vi "PSTRA-Init Reanalysis.vi"(0 "Path":path, 5 "PSTR Params":T31={"Stimulus"={"Ear"=enum."Right", "BW (oct)"=0.0, "Seed"=0, "Ramp (ms)"=0.0, "On time (ms)"=0.0, "Off time (ms)"=0.0, "Delay (ms)"=10000.0}, "FreqSeq"={"Min (kHz)"=0.0, "Max (kHz)"=0.0, "Step (oct)"=0.0}, "LevelSeq"={"Min (dB)"=0.0, "Max (dB)"=0.0, "Step (dB)"=0.0}, "Seq"={"Order"=enum."Sequential", "Averages"=0}, "Response"={"Grass gain"=0.0, "Window (ms)"=0.0}, "Hidden"={"Sample rate (Hz)"=0.0, "Nfft"=0, "save raw"=FALSE, "sep"=0.0, "Window"=enum."NONE"}, "RejThr"=0.0}) -> (4 "Data":T28, 8 "SCL":T27[](array[typedef]), 14 "Runtime out":T1 {"window" items=["None ", "Hanning", "Hamming", "Blackman-Harris", "Exact Blackman", "Blackman", "Flat Top", "4 Term B-Harris ", "7 Term B-Harris", "Low Sidelobe"]; "stimChan"."Filter"."Stages"."IIR Filter"."Forward Coefficients" format="%.4f"; "stimChan"."Filter"."Stages"."IIR Filter"."Reverse Coefficients" format="%.4f"})   [LabVIEW 2020]
uses:
  PSTR VIs/Typedefs/PSTR-Parameters.ctl
  PSTR VIs/Typedefs/PSTR-Stimulus Params.ctl
  Utility VIs/Type Defs/Left-Right ring.ctl
  PSTR VIs/Typedefs/PSTR-FreqSeq Params.ctl
  PSTR VIs/Typedefs/PSTR-LevelSeq Params.ctl
  PSTR VIs/Typedefs/PSTR-SeqParams.ctl
  PSTR VIs/Typedefs/PSTR-Response Params.ctl
  PSTR VIs/Typedefs/PSTR-Hidden Params.ctl
  PSTR VIs/Typedefs/PSTR-Window Shape.ctl
  PSTR VIs/Typedefs/PSTR-Data.ctl
  PSTR VIs/Typedefs/PSTR-Model Fit.ctl
  PSTR VIs/Typedefs/PSTR-Fit Parameters.ctl
  Typedefs/PSTR-SCL Element.ctl
  PSTR VIs/Typedefs/PSTR-Runtime Data.ctl
  Signal Synthesis VIs/Controls/Stimulus Channel (Full)/Full Stimulus Channel Data.ctl
  Signal Synthesis VIs/Controls/Waveform XCtl/Waveform Data.ctl
  Signal Synthesis VIs/Controls/Waveform XCtl/Waveform Enum.ctl
  Signal Synthesis VIs/Waveform VIs/Tone VIs/Tone Params.ctl
  Signal Synthesis VIs/Waveform VIs/Pulse Train VIs/Pulse Train Params.ctl
  Signal Synthesis VIs/Waveform VIs/Pulse Train VIs/Pulse Polarity.ctl
  Signal Synthesis VIs/Waveform VIs/Pulse Train VIs/PT-Continuous State.ctl
  Signal Synthesis VIs/Waveform VIs/Noise VIs/Noise Params.ctl
  Signal Synthesis VIs/Waveform VIs/File VIs/StimFile-Params.ctl
  Signal Synthesis VIs/Waveform VIs/FM Sweep VIs/FM Sweep Params.ctl
  Signal Synthesis VIs/Waveform VIs/Chirp Train VIs/Chirp Train.ctl
  Signal Synthesis VIs/Waveform VIs/Chirp Train VIs/Chirp Train Params.ctl
  Signal Synthesis VIs/Waveform VIs/Complex Tone VIs/CT-Params.ctl
  Signal Synthesis VIs/Waveform VIs/Complex Tone VIs/CT-Phase Enum.ctl
  Signal Synthesis VIs/Waveform VIs/Complex Tone VIs/CT-Runtime Data.ctl
  Signal Synthesis VIs/Waveform VIs/Moving Ripple VIs/Moving Ripple.ctl
  Signal Synthesis VIs/Waveform VIs/Moving Ripple VIs/Moving Ripple.Params.ctl
  Signal Synthesis VIs/Waveform VIs/Moving Ripple VIs/Moving Ripple.Data.ctl
  Signal Synthesis VIs/Controls/Advanced Filter XCtl/Filter Data.ctl
  Signal Synthesis VIs/Filter VIs/Filter-Bandwidth Units.ctl
  Signal Synthesis VIs/Controls/Burst XCtl/Burst Data.ctl
  Signal Synthesis VIs/Controls/Level XCtl/Level Data.ctl
  Signal Synthesis VIs/Controls/Level XCtl/Level Units.ctl
  Signal Synthesis VIs/Controls/Advanced Options XCtl/Advanced Stimulus Options.ctl
  Signal Synthesis VIs/Modulation VIs/SAM VIs/SAM Params.ctl
  Signal Synthesis VIs/Controls/Waveform XCtl/Waveform XCtl.xctl
  Signal Synthesis VIs/Controls/Advanced Filter XCtl/Advanced Filter XCtl.xctl
  Signal Synthesis VIs/Controls/Burst XCtl/Burst Control.xctl
  Signal Synthesis VIs/Controls/Level XCtl/Level XCtl.xctl
  Signal Synthesis VIs/Controls/Advanced Options XCtl/Advanced Stimulus Options.xctl
  Signal Synthesis VIs/Controls/Stimulus Channel (Full)/Stimulus Channel (Full).xctl
panel:
  # "NF x NL x 2 x Npts"
  # "NF x NL x Npts"
  # "NF x NL"
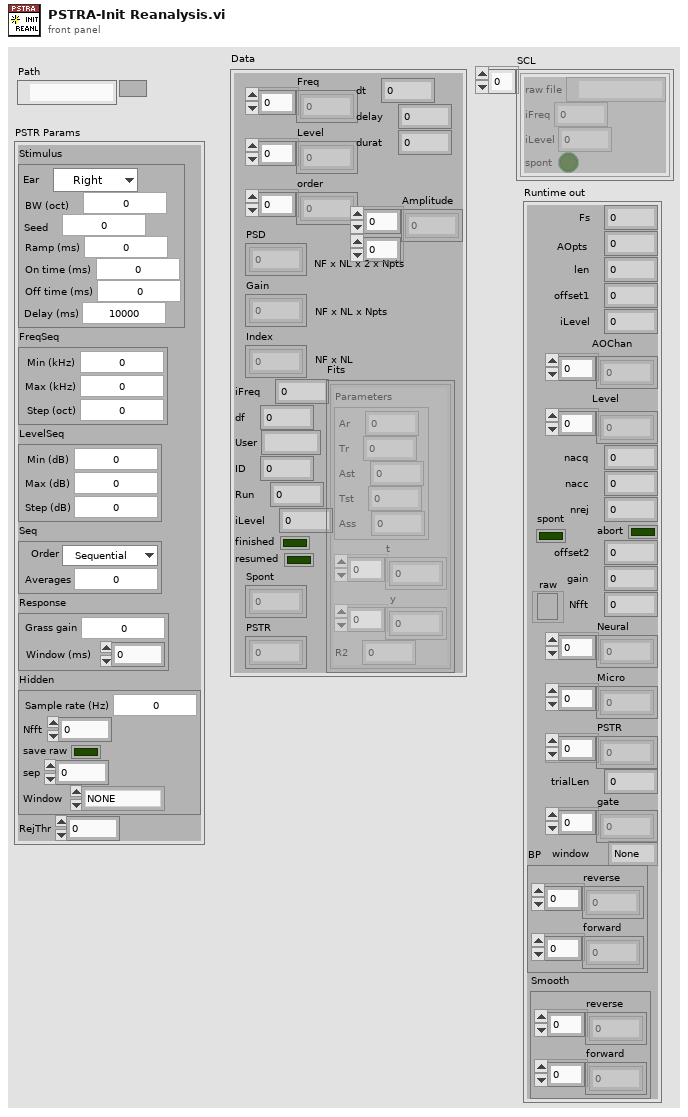
[diagram p1: front panel]
types:
  T1 = typedef "PSTR-Runtime Data.ctl" = cluster{"Fs":dbl, "AOpts":i32, "stimChan":T2, "len":i32, "offset1":i32, "iLevel":i32, "AOChan":i32[], "Level":dbl[], "nacc":i32, "nrej":i32, "nacq":i32, "abort":bool, "offset2":i32, "gain":dbl, "Nfft":i32, "Neural":dbl[], "Micro":dbl[], "raw":refnum<file>, "spont":bool, "PSTR":dbl[], "trialLen":i32, "gate":dbl[], "window":u16, "BP":cluster{"reverse":dbl[], "forward":dbl[]}, "Smooth":cluster{"reverse":dbl[], "forward":dbl[]}}
  T2 = typedef "Stimulus Channel (Full).xctl/Full Stimulus Channel Data.ctl" = cluster{"Waveform":T3, "Filter":T20, "Burst":T22, "Level":T23, "Name":string, "Advanced":T25, "SAM":T26}
  T3 = typedef "Waveform XCtl.xctl/Waveform Data.ctl" = cluster{"Type":T4, "Tone":T5, "Pulse Train":T6, "Noise":T9, "File":T10, "FMSweep":T11, "Chirp Train":T12, "Complex Tone":cluster{"Params":T14, "Data":T16}, "Moving Ripple":T17}
  T4 = typedef "Waveform Enum.ctl" = enum16{"OFF", "Tone", "Noise", "Pulse Train", "File", "FM Sweep", "Chirp Train", "Complex Tone", "FM Tone", "Moving Ripple"}
  T5 = typedef "Tone Params.ctl" = cluster{"Frequency (kHz)":dbl, "Last Freq":dbl, "Last Phase":dbl}
  T6 = typedef "Pulse Train Params.ctl" = cluster{"Pulse width (us)":dbl, "Pulse rate (Hz)":dbl, "Gap (ms)":dbl, "Polarity":T7, "PT State":T8, "Asynch":bool}
  T7 = typedef "Pulse Polarity.ctl" = enum16{"POS", "NEG", "POS-NEG", "NEG-POS"}
  T8 = typedef "PT-Continuous State.ctl" = cluster{"Template":dbl[], "Nperiod":i32, "Index":i32, "Pulse Rate (Hz)":dbl, "Phase (cycles)":dbl, "Noff":i32}
  T9 = typedef "Noise Params.ctl" = cluster{"InvFilt":bool, "Noise":dbl[], "CurPt":i32, "Aweight":bool, "Seed":i32, "afile":path}
  T10 = typedef "StimFile-Params.ctl" = cluster{"Filename":path, "Signal":dbl[], "Channel":i32, "stream":bool, "offset":i32, "nreps":i32, "loops":i32, "Randomize":bool, "order":i32[], "Seed":i32, "Tokens":i32}
  T11 = typedef "FM Sweep Params.ctl" = cluster{"Rate (oct/s)":dbl, "Fmin (Hz)":dbl, "Fmax (Hz)":dbl, "Ramp (ms)":dbl, "Linear":bool}
  T12 = typedef "Chirp Train.ctl" = cluster{"Params":T13, "Data":cluster{"WF":dbl[]}}
  T13 = typedef "Chirp Train Params.ctl" = cluster{"Fmin (kHz)":dbl, "Fmax (kHz)":dbl, "Compensate":bool, "Duration (ms)":dbl}
  T14 = typedef "CT-Params.ctl" = cluster{"F0 (Hz)":dbl, "Band":cluster{"Flow (Hz)":dbl, "Fhigh (Hz)":dbl}, "Phase":T15, "Min F0 (Hz)":dbl, "Max F0 (Hz)":dbl, "ContinRandPhase":bool, "Max peak factor":dbl, "Max mod depth":dbl, "MinHarmNum":i32, "MaxHarmNum":i32, "Level Mode":enum16{"per component", "overall rms"}, "% jitter":dbl}
  T15 = typedef "CT-Phase Enum.ctl" = enum16{"Cosine", "Random", "Alternating"}
  T16 = typedef "CT-Runtime Data.ctl" = cluster{"Ncomp":i32, "MinHarm":i32, "Phase":dbl[], "Amplitude":dbl[], "Npts/frame":i32, "Last F0":dbl, "Fmin":dbl, "Fmax":dbl, "Lslope":dbl, "randphase":bool, "overall rms":bool, "fmult":dbl[], "jittered":bool}
  T17 = typedef "Moving Ripple.ctl" = cluster{"Params":T18, "Data":T19}
  T18 = typedef "Moving Ripple.Params.ctl" = cluster{"Fmin":dbl, "Fmax":dbl, "Density":dbl, "Velocity":dbl, "Depth":dbl, "Phase":dbl, "Comp/oct":i32}
  T19 = typedef "Moving Ripple.Data.ctl" = cluster{"Freq":dbl[], "A":dbl[], "phase":dbl[], "Phase":dbl}
  T20 = typedef "Advanced Filter XCtl.xctl/Filter Data.ctl" = cluster{"Type":enum16{"Lowpass", "Highpass", "Bandpass", "Bandstop", "OFF"}, "CF (kHz)":dbl, "BW (kHz)":dbl, "Cascade":bool, "Quadrature":bool, "Scale Factor":dbl, "Stages":cluster{"IIR Filter":cluster{"filter structure":enum32{"IIR 2nd Order", "IIR 4th Order"}, "Reverse Coefficients":dbl[], "Forward Coefficients":dbl[]}, "State":dbl[]}[], "Class":enum16{"Elliptic", "Butterworth"}, "Order":i32, "BWUnits":T21}
  T21 = typedef "Filter-Bandwidth Units.ctl" = enum16{"Linear", "Octaves", "Min-Max"}
  T22 = typedef "Burst Control.xctl/Burst Data.ctl" = cluster{"Active":bool, "Delay (ms)":dbl, "Duration (ms)":dbl, "Ramp (ms)":dbl, "Rate (Hz)":dbl, "Trepeat (ms)":dbl, "Repeat":bool}
  T23 = typedef "Level XCtl.xctl/Level Data.ctl" = cluster{"Level":dbl, "Units":T24, "Max":dbl, "Multiplier":dbl, "Cal File":path, "Cal":cluster{"Freq (Hz)":dbl[], "Mag (dB SPL)":dbl[], "Phase (deg)":dbl[]}}
  T24 = typedef "Level Units.ctl" = enum16{"dB atten", "dB SPL", "dB re 1 Vrms", "dB V/Hz½", "mW", "dB HL", "Volts", "dB mW"}
  T25 = typedef "Advanced Stimulus Options.xctl/Advanced Stimulus Options.ctl" = cluster{"Rep Mask":string, "AltPol":bool, "Var":string, "Expr":string, "Persist":bool}
  T26 = typedef "SAM Params.ctl" = cluster{"Active":bool, "Frequency (Hz)":dbl, "Depth":dbl, "Init Phase (cycles)":dbl, "phase (degrees)":dbl, "Asynch":bool}
  T27 = typedef "PSTR-SCL Element.ctl" = cluster{"raw file":path, "iFreq":i32, "iLevel":i32, "spont":bool}
  T28 = typedef "PSTR-Data.ctl" = cluster{"Freq":dbl[], "Level":dbl[], "order":i32[], "PSD":dbl[][][][], "Gain":dbl[][][], "Index":dbl[][], "iFreq":i32, "df":dbl, "User":string, "ID":i32, "Run":i32, "iLevel":i32, "finished":bool, "resumed":bool, "Spont":dbl[][], "PSTR":dbl[][][], "dt":dbl, "delay":dbl, "durat":dbl, "Fits":T29[][], "Amplitude":dbl[][]}
  T29 = typedef "PSTR-Model Fit.ctl" = cluster{"Parameters":T30, "t":dbl[], "y":dbl[], "R2":dbl}
  T30 = typedef "PSTR-Fit Parameters.ctl" = cluster{"Ar":dbl, "Tr":dbl, "Ast":dbl, "Tst":dbl, "Ass":dbl}
  T31 = typedef "PSTR-Parameters.ctl" = cluster{"Stimulus":T32, "FreqSeq":T34, "LevelSeq":T35, "Seq":T36, "Response":T37, "Hidden":T38, "RejThr":dbl}
  T32 = typedef "PSTR-Stimulus Params.ctl" = cluster{"Ear":T33, "BW (oct)":dbl, "Seed":i32, "Ramp (ms)":dbl, "On time (ms)":dbl, "Off time (ms)":dbl, "Delay (ms)":dbl}
  T33 = typedef "Left-Right ring.ctl" = enum16{"Right", "Left"}
  T34 = typedef "PSTR-FreqSeq Params.ctl" = cluster{"Min (kHz)":dbl, "Max (kHz)":dbl, "Step (oct)":dbl}
  T35 = typedef "PSTR-LevelSeq Params.ctl" = cluster{"Min (dB)":dbl, "Max (dB)":dbl, "Step (dB)":dbl}
  T36 = typedef "PSTR-SeqParams.ctl" = cluster{"Order":enum16{"Sequential", "Random"}, "Averages":i32}
  T37 = typedef "PSTR-Response Params.ctl" = cluster{"Grass gain":dbl, "Window (ms)":dbl}
  T38 = typedef "PSTR-Hidden Params.ctl" = cluster{"Sample rate (Hz)":dbl, "Nfft":i32, "save raw":bool, "sep":dbl, "Window":T39}
  T39 = typedef "PSTR-Window Shape.ctl" = enum16{"NONE", "Hamming"}
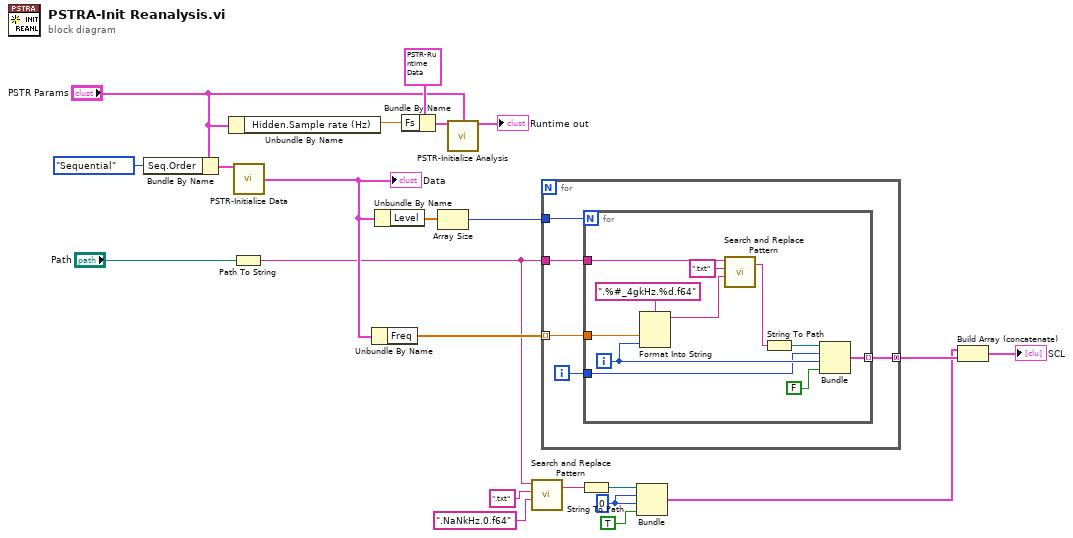
[diagram p0: block diagram]
diagram:
  w3 = 0
  n1 = Bundle By Name(cluster="PSTR Params", "Seq.Order"=enum16{"Sequential", "Random"}."Sequential") -> (w20:T31)
  n2 = Unbundle By Name("PSTR Params") -> ("Hidden.Sample rate (Hz)"=w10:dbl)
  n3 = Path To String(path="Path") -> (string=w8:string)
  n4 = call "PSTR-Initialize Data.vi"("PSTR Params"=w20) -> ("Data"=w15:T28)  [unwired: 13 in, 1 out]
  "Data" <- w15
  n5 = Unbundle By Name(w15) -> ("Freq"=w22:dbl[])
  n6 = Unbundle By Name(w15) -> ("Level"=w18:dbl[])
  n7 = Bundle By Name(cluster=T1 {"Fs"=0.0, "AOpts"=0, "stimChan"={"Waveform"={"Type"=enum."Tone", "Tone"={"Frequency (kHz)"=0.0, "Last Freq"=0.0, "Last Phase"=0.0}, "Pulse Train"={"Pulse width (us)"=0.0, "Pulse rate (Hz)"=0.0, "Gap (ms)"=0.0, "Polarity"=enum."POS", "PT State"={"Template"=[], "Nperiod"=0, "Index"=0, "Pulse Rate (Hz)"=0.0, "Phase (cycles)"=0.0, "Noff"=0}, "Asynch"=FALSE}, "Noise"={"InvFilt"=FALSE, "Noise"=[], "CurPt"=0, "Aweight"=FALSE, "Seed"=0, "afile"=path ""}, "File"={"Filename"=path "", "Signal"=[], "Channel"=0, "stream"=FALSE, "offset"=0, "nreps"=0, "loops"=0, "Randomize"=FALSE, "order"=[], "Seed"=0, "Tokens"=0}, "FMSweep"={"Rate (oct/s)"=0.0, "Fmin (Hz)"=0.0, "Fmax (Hz)"=0.0, "Ramp (ms)"=0.0, "Linear"=FALSE}, "Chirp Train"={"Params"={"Fmin (kHz)"=4.0, "Fmax (kHz)"=64.0, "Compensate"=FALSE, "Duration (ms)"=2.0}, "Data"={"WF"=[]}}, "Complex Tone"={"Params"={"F0 (Hz)"=0.0, "Band"={"Flow (Hz)"=0.0, "Fhigh (Hz)"=0.0}, "Phase"=enum."Cosine", "Min F0 (Hz)"=0.0, "Max F0 (Hz)"=0.0, "ContinRandPhase"=FALSE, "Max peak factor"=inf, "Max mod depth"=2.0, "MinHarmNum"=0, "MaxHarmNum"=0, "Level Mode"=enum."per component", "% jitter"=0.0}, "Data"={"Ncomp"=0, "MinHarm"=0, "Phase"=[], "Amplitude"=[], "Npts/frame"=0, "Last F0"=0.0, "Fmin"=0.0, "Fmax"=0.0, "Lslope"=0.0, "randphase"=FALSE, "overall rms"=FALSE, "fmult"=[], "jittered"=FALSE}}, "Moving Ripple"={"Params"={"Fmin"=0.0, "Fmax"=0.0, "Density"=0.0, "Velocity"=0.0, "Depth"=0.0, "Phase"=0.0, "Comp/oct"=0}, "Data"={"Freq"=[], "A"=[], "phase"=[], "Phase"=0.0}}}, "Filter"={"Type"=enum."Lowpass", "CF (kHz)"=0.0, "BW (kHz)"=0.0, "Cascade"=FALSE, "Quadrature"=FALSE, "Scale Factor"=0.0, "Stages"=[], "Class"=enum."Elliptic", "Order"=0, "BWUnits"=enum."Linear"}, "Burst"={"Active"=FALSE, "Delay (ms)"=0.0, "Duration (ms)"=0.0, "Ramp (ms)"=0.0, "Rate (Hz)"=0.0, "Trepeat (ms)"=0.0, "Repeat"=FALSE}, "Level"={"Level"=0.0, "Units"=enum."dB atten", "Max"=0.0, "Multiplier"=0.0, "Cal File"=path "", "Cal"={"Freq (Hz)"=[], "Mag (dB SPL)"=[], "Phase (deg)"=[]}}, "Name"="", "Advanced"={"Rep Mask"="", "AltPol"=FALSE, "Var"="", "Expr"="", "Persist"=FALSE}, "SAM"={"Active"=FALSE, "Frequency (Hz)"=0.0, "Depth"=0.0, "Init Phase (cycles)"=0.0, "phase (degrees)"=0.0, "Asynch"=FALSE}}, "len"=0, "offset1"=0, "iLevel"=0, "AOChan"=[], "Level"=[], "nacc"=0, "nrej"=0, "nacq"=0, "abort"=FALSE, "offset2"=0, "gain"=0.0, "Nfft"=0, "Neural"=[], "Micro"=[], "raw"=refnum, "spont"=FALSE, "PSTR"=[], "trialLen"=0, "gate"=[], "window"=0, "BP"={"reverse"=[], "forward"=[]}, "Smooth"={"reverse"=[], "forward"=[]}} ("Runtime in"), "Fs"=w10) -> (w11:T1)
  n8 = Array Size(array=w18) -> (size(s)=w17:i32)
  n9 = call "PSTR-Initialize Analysis.vi"("Runtime in"=w11, "PSTR Params"="PSTR Params") -> ("Runtime out"=→"Runtime out":T1)  [unwired: 12 in, 1 out]
  n10 = call <vilib>:"Search and Replace Pattern.vi"("string"=w8, "regular expression (\"\")"=".txt" ("regular expression (\"\")"), "replace string (\"\")"=".NaNkHz.0.f64" ("format string")) -> ("result string"=w4:string)  [unwired: 2 in, 1 out]
  n11 = for {
    tunnel: w22 -> [w27] mode=indexing
    tunnel: w8 -> [w26]
    tunnel: w17 -> [w25]
    tunnel: [w23] -> w16 mode=concatenating
    i -> [w24]
    n12 = for {
      N: w25 -> [_]
      tunnel: w27 -> [w37]
      tunnel: w26 -> [w36]
      tunnel: w24 -> [w30]
      tunnel: [w29] -> w23 mode=indexing
      i -> [w33]
      n13 = Format Into String(format string=".%#_4gkHz.%d.f64", w37, w33) -> (resulting string=w34:string)  [unwired: 2 in, 1 out]
      n14 = call <vilib>:"Search and Replace Pattern.vi"("string"=w36, "regular expression (\"\")"=".txt" ("regular expression (\"\")"), "replace string (\"\")"=w34) -> ("result string"=w32:string)  [unwired: 2 in, 1 out]
      n15 = String To Path(string=w32) -> (path=w31:path)
      n16 = Bundle(w31, w30, w33, FALSE) -> (w29:cluster{path, i32, i32, bool})  [unwired: 1 in]
    }
  }
  n17 = String To Path(string=w4) -> (path=w6:path)
  n18 = Bundle(w6, w3, w3, TRUE) -> (w1:cluster{path, i32, i32, bool})  [unwired: 1 in]
  n19 = Build Array (concatenate)(w1, w16) -> (→"SCL":cluster{path, i32, i32, bool}[])
